vi "RichToFlatsift_proxy_v1_CreateLabviewIngestionConfigRequest.vi"(5 "OutputClusterType":T1, 11 "InputCluster":T6) -> (3 "OutputCluster":T1)   [LabVIEW 2024, in "SiftProxy_client.lvlib"]
uses:
  SiftProxy_client.lvlib
  sift_proxy_v1_CreateLabviewIngestionConfigRequest.ctl
  sift_proxy_v1_ChannelConfig.ctl
  sift_proxy_v1_ChannelDataType.ctl
  sift_proxy_v1_ChannelEnumType.ctl
  sift_proxy_v1_ChannelBitFieldElement.ctl
  sift_proxy_v1_CreateLabviewIngestionConfigRequest_Flat.ctl
  sift_proxy_v1_ChannelConfig_Flat.ctl
  sift_proxy_v1_ChannelEnumType_Flat.ctl
  sift_proxy_v1_ChannelBitFieldElement_Flat.ctl
  RichToFlatsift_proxy_v1_ChannelEnumType.vi
  RichToFlatsift_proxy_v1_ChannelBitFieldElement.vi
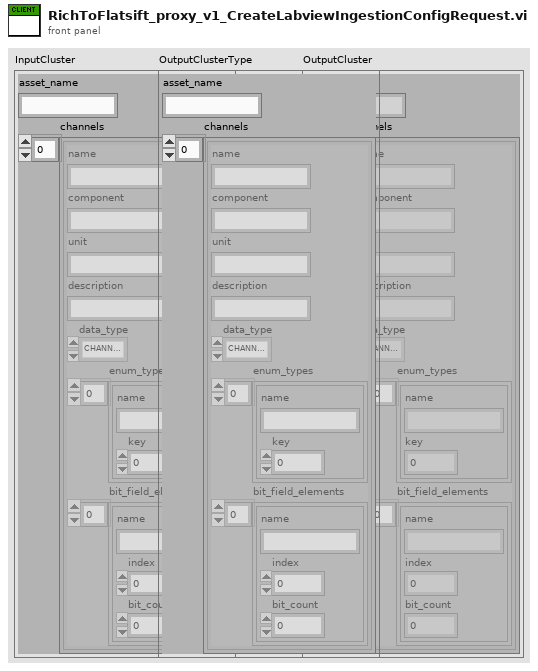
[diagram p1: front panel]
types:
  T1 = typedef "SiftProxy_client.lvlib/sift_proxy_v1_CreateLabviewIngestionConfigRequest_Flat.ctl" = cluster{"asset_name":string, "channels":T2[]}
  T2 = typedef "SiftProxy_client.lvlib/sift_proxy_v1_ChannelConfig_Flat.ctl" = cluster{"name":string, "component":string, "unit":string, "description":string, "data_type":T3, "enum_types":T4[], "bit_field_elements":T5[]}
  T3 = typedef "SiftProxy_client.lvlib/sift_proxy_v1_ChannelDataType.ctl" = enum32{"CHANNEL_DATA_TYPE_UNSPECIFIED", "CHANNEL_DATA_TYPE_DOUBLE", "CHANNEL_DATA_TYPE_STRING", "CHANNEL_DATA_TYPE_ENUM", "CHANNEL_DATA_TYPE_BIT_FIELD", "CHANNEL_DATA_TYPE_BOOL", "CHANNEL_DATA_TYPE_FLOAT", "CHANNEL_DATA_TYPE_INT_32", "CHANNEL_DATA_TYPE_UINT_32", "CHANNEL_DATA_TYPE_INT_64", "CHANNEL_DATA_TYPE_UINT_64"}
  T4 = typedef "SiftProxy_client.lvlib/sift_proxy_v1_ChannelEnumType_Flat.ctl" = cluster{"name":string, "key":u32}
  T5 = typedef "SiftProxy_client.lvlib/sift_proxy_v1_ChannelBitFieldElement_Flat.ctl" = cluster{"name":string, "index":i32, "bit_count":u32}
  T6 = typedef "SiftProxy_client.lvlib/sift_proxy_v1_CreateLabviewIngestionConfigRequest.ctl" = cluster{"asset_name":string, "channels":T7[]}
  T7 = typedef "SiftProxy_client.lvlib/sift_proxy_v1_ChannelConfig.ctl" = cluster{"name":string, "component":string, "unit":string, "description":string, "data_type":T3, "enum_types":T8[], "bit_field_elements":T9[]}
  T8 = typedef "SiftProxy_client.lvlib/sift_proxy_v1_ChannelEnumType.ctl" = cluster{"name":string, "key":u32}
  T9 = typedef "SiftProxy_client.lvlib/sift_proxy_v1_ChannelBitFieldElement.ctl" = cluster{"name":string, "index":i32, "bit_count":u32}
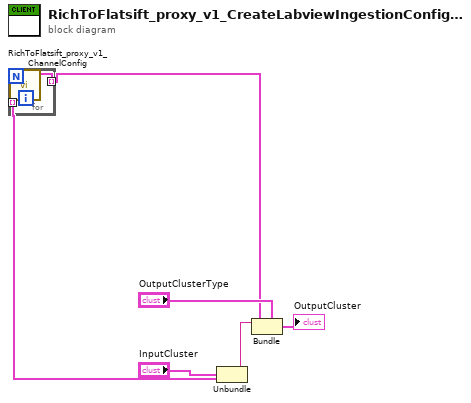
[diagram p0: block diagram]
diagram:
  n1 = Unbundle "Unbundle"("InputCluster") -> ("asset_name"=w3:string, "channels"=w2:T7[])
  n2 = for {
    tunnel: w2 -> [w8] mode=indexing
    tunnel: [w7] -> w1 mode=indexing
    n3 = call "RichToFlatsift_proxy_v1_ChannelConfig.vi"("InputCluster"=w8) -> ("OutputCluster"=w7:T2)  [unwired: 10 in]
  }
  n4 = Bundle "Bundle"(cluster="OutputClusterType", "asset_name"=w3, "channels"=w1) -> (→"OutputCluster":T1)
